vi "Set Printer Settings.vi"(10 "Array":refnum<vi>[](array[refnum]), 11 "VI in":refnum<vi>) -> ()   [LabVIEW 2013]
uses:
  <vilib>/Utility/miscctls.llb/LVPrintingMarginsTypeDef.ctl
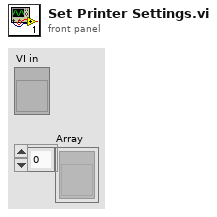
[diagram p1: front panel]
types:
  T1 = typedef "LVPrintingMarginsTypeDef.ctl" = cluster{"Top":sgl, "Left":sgl, "Bottom":sgl, "Right":sgl, "Measurement System":enum8{"Inches", "cm"}}
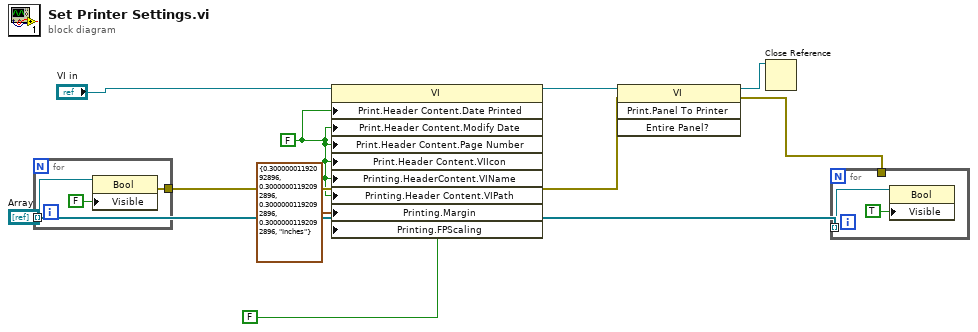
[diagram p0: block diagram]
diagram:
  w3 = FALSE
  n1 = for {
    tunnel: "Array" -> [w12] mode=indexing
    tunnel: [w10] -> w9
    n2 = property class="Bool"(reference=w12, "Visible"=FALSE) -> (error out=w10:errorcluster)  [unwired: 1 in, 1 out]
  }
  n3 = property class="VI"(reference="VI in", "Print.Header Content.Date Printed"=w3, "Print.Header Content.Modify Date"=w3, "Print.Header Content.Page Number"=w3, "Print.Header Content.VIIcon"=w3, "Printing.HeaderContent.VIName"=w3, "Printing.Header Content.VIPath"=w3, "Printing.Margin"=T1 {"Top"=0.3, "Left"=0.3, "Bottom"=0.3, "Right"=0.3, "Measurement System"=enum."Inches"} ("Printing:Margins"), "Printing.FPScaling"=FALSE ("Printing:Front Panel Scaling?")) -> (reference out=w4:refnum<vi>)  [unwired: 1 in, 1 out]
  n4 = invoke class="VI" method="Print.Panel To Printer"(reference=w4, error in=w9) -> (reference out=w6:refnum<vi>, error out=w7:errorcluster)  [unwired: 2 in, 2 out]
  n5 = Close Reference(reference=w6) -> ()  [unwired: 1 in, 1 out]
  n6 = for {
    tunnel: "Array" -> [w14] mode=indexing
    tunnel: w7 -> [_]
    n7 = property class="Bool"(reference=w14, "Visible"=TRUE) -> ()  [unwired: 1 in, 2 out]
  }
